vi "Keithley 230 V prop B^2.vi"(2 "Point #":i32, 3 "GPIB Data In":dbl[](array[numeric]) format="%.2e", 5 "Instrument Address":refnum<visa-resource-name>) -> (0 "Stop":bool, 1 "Keithley 230 Voltage":dbl[](array[numeric]) format="%.2e")   [LabVIEW 2024]
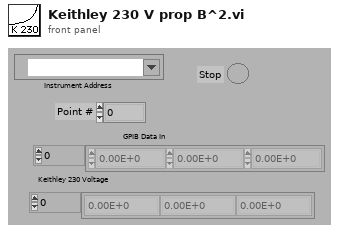
[diagram p1: front panel]
types:
  T1 = cluster{"Instrument":string, "ID Test String":string, "Terminator Character":string, u32, bool}
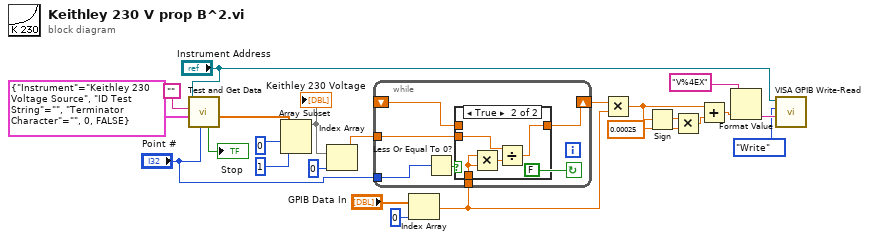
[diagram p0: block diagram]
diagram:
  n1 = call "Test and Get Data.vi"("Point #"="Point #", "Instrument Info"=T1 {"Instrument"="Keithley 230 Voltage Source", "ID Test String"="", "Terminator Character"="", 0, FALSE}, "Command String"="", "VISA Sesson"="Instrument Address") -> ("Measurement"=w5:dbl[], "Stop"=→"Stop":bool)  [unwired: 2 in, 3 out]
  n2 = Array Subset(array=w5, index=0, length=1) -> (w21:dbl[])
  "Keithley 230 Voltage" <- w21
  n3 = Index Array(array=w21, index=0) -> (element=w13:dbl)
  n4 = Index Array(array="GPIB Data In", index=0) -> (element=w8:dbl)
  n5 = while {
    tunnel: "Point #" -> [w24]
    tunnel: w8 -> [w26]
    tunnel: w13 -> [w27]
    shift-left: _ -> [w29]
    shift-right: [w28] -> w14
    stop <- FALSE continue-if-true
    n6 = Less Or Equal To 0?(x=w24) -> (x <= 0?=w30:bool)
    n7 = case shown="True" w30 {
      tunnel: w29 -> [w31 _]
      tunnel: [w31 w32] -> w28
      tunnel: w27 -> [_ w34]
      tunnel: w26 -> [_ w33]
      frame False {
      }
      frame True {
        n8 = Multiply(x=w33, y=w33) -> (x*y=w35:dbl)
        n9 = Divide(x=w34, y=w35) -> (x/y=w32:dbl)
      }
    }
  }
  n10 = Multiply(x=w14, y=w8) -> (x*y=w18:dbl)
  n11 = Sign(1:w18) -> (0:w19:dbl)
  n12 = Multiply(x=w19, y=0.00025) -> (x*y=w17:dbl)
  n13 = Add(x=w18, y=w17) -> (x+y=w16:dbl)
  n14 = Format Value(format string="V%4EX", value (0)=w16) -> (output string=w7:string)  [unwired: 1 in]
  n15 = call "VISA GPIB Write-Read.vi"("Command"=w7, "Action"=enum16{"Write", "Read", "Write & Read"}."Write", "VISA resource name"="Instrument Address") -> ()  [unwired: 5 in, 4 out]
